vi "Initialize.vi"(8 "error in (no error)":errorcluster, 9 "Baud Rate":u32(ring)=9600 items=["9600"=9600, "38400"=38400, "57600"=57600, "19200"=19200], 11 "VISA resource name":refnum<visa-resource-name>) -> (0 "error out":errorcluster, 3 "VISA resource name out":refnum<visa-resource-name>)   [LabVIEW 2010, in "FEM-03.lvlib"]
doc: "Establishes communication with the instrument and optionally performs an instrument identification query and/or an instrument reset. It also places the instrument in a default state needed for other instrument driver operations. Therefore, call this VI before calling other instrument driver VIs for this instrument. Generally, you need to call the Initialize VI only once at the beginning of an application."
uses:
  FEM-03.lvlib
panel:
  # "(c) 2007 <Enter Company Name Here>.  ALL RIGHTS RESERVED."
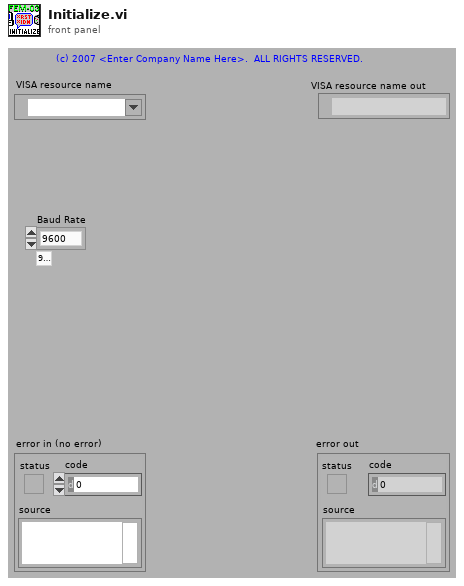
[diagram p1: front panel]
types:
  T1 = cluster{"Baud Rate":u32, "Parity":u16, "Data Bits":u16, "Stop Bits":u16, "Flow Control":u16}
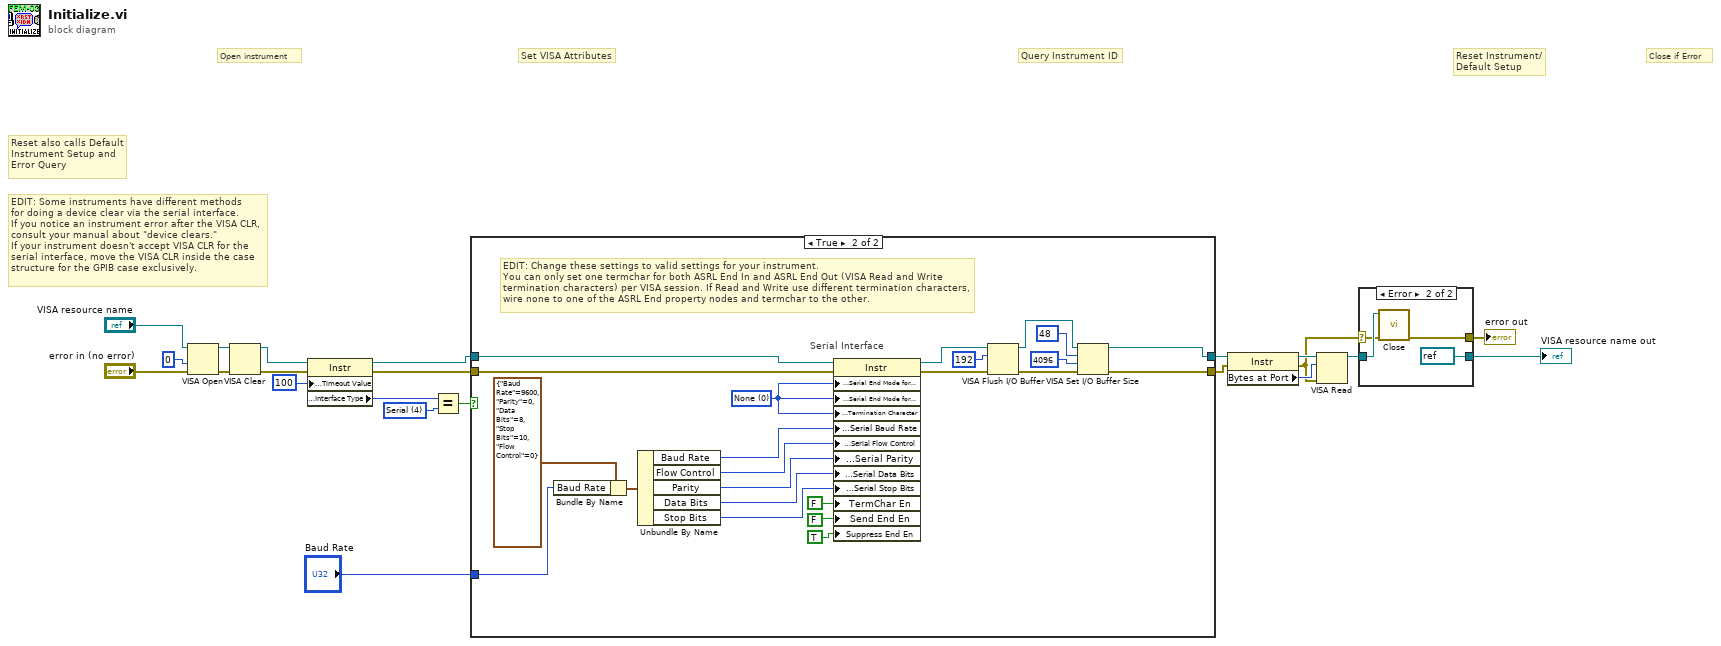
[diagram p0: block diagram]
diagram:
  w15 = u16 4 items=["GPIB"=1, "VXI"=2, "GPIB-VXI"=3, "Serial"=4, "PXI"=5, "TCPIP"=6, "USB"=7] ("Interface Information:Interface Type")
  # "Reset also calls Default Instrument Setup and Error Query"
  # "EDIT: Some instruments have different methods\nfor doing a device clear via the serial interface.  \nIf you notice an instrument error after the VISA CLR,\nconsult your manual about \"device clears.\"  \nIf your instrument doesn't accept VISA CLR for the\nserial interface, move the VISA CLR inside the case \nstructure for the GPIB case exclusively."
  # "Set VISA Attributes"
  # "Close if Error"
  # "Query Instrument ID"
  # "Reset Instrument/\nDefault Setup"
  # "Open instrument"
  n1 = VISA Open(access mode=u32 0, error in (no error)="error in (no error)", VISA resource name="VISA resource name") -> (VISA resource name=w13:refnum<visa-resource-name>, error out=w12:errorcluster)  [unwired: 2 in]
  n2 = VISA Clear(VISA resource name=w13, error in (no error)=w12) -> (VISA resource name out=w11:refnum<visa-resource-name>, error out=w10:errorcluster)
  n3 = property class="Instr"(reference=w11, error in=w10, "General Settings:Timeout Value"=u32 100) -> (reference out=w18:refnum<visa-resource-name>, error out=w17:errorcluster, "Interface Information:Interface Type"=w20:u16)
  n4 = Equal?(x=w20, y=w15) -> (x = y?=w16:bool)
  n5 = case shown="True" w16 {
    tunnel: [w23 w44] -> w6
    tunnel: [w24 w41] -> w3
    tunnel: w18 -> [w23 w46]
    tunnel: w17 -> [w24 w47]
    tunnel: "Baud Rate" -> [_ w25]
    frame False {
      # "EDIT: Remove interfaces not\nsupported by your instrument."
      # "GPIB, TCP/IP, and USB Interface"
    }
    frame True {
      w27 = u16 0 items=["None", "LastBit", "TermChar"] ("Serial Settings:Serial End Mode for Reads")
      # "EDIT: Change these settings to valid settings for your instrument.\nYou can only set one termchar for both ASRL End In and ASRL End Out (VISA Read and Write termination characters) per VISA session. If Read and Write use different termination characters, wire none to one of the ASRL End property nodes and termchar to the other."
      # "Serial Interface"
      n6 = Bundle By Name(cluster=T1 {"Baud Rate"=9600, "Parity"=0, "Data Bits"=8, "Stop Bits"=10, "Flow Control"=0} ("Serial Configuration"), "Baud Rate"=w25) -> (w26:T1)
      n7 = Unbundle By Name(w26) -> ("Baud Rate"=w36:u32, "Flow Control"=w32:u16, "Parity"=w34:u16, "Data Bits"=w35:u16, "Stop Bits"=w31:u16)
      n8 = property class="Instr"(reference=w46, error in=w47, "Serial Settings:Serial End Mode for Reads"=w27, "Serial Settings:Serial End Mode for Writes"=w27, "Message Based Settings:Termination Character"=w27, "Serial Settings:Serial Baud Rate"=w36, "Serial Settings:Serial Flow Control"=w32, "Serial Settings:Serial Parity"=w34, "Serial Settings:Serial Data Bits"=w35, "Serial Settings:Serial Stop Bits"=w31, "TermChar En"=FALSE ("Message Based Settings:Termination Character Enable"), "Send End En"=FALSE ("Message Based Settings:Send End Enable"), "Suppress End En"=TRUE ("Message Based Settings:Suppress End Enable")) -> (reference out=w40:refnum<visa-resource-name>, error out=w43:errorcluster)
      n9 = VISA Flush I/O Buffer(VISA resource name=w40, mask (16)=u16 192, error in (no error)=w43) -> (VISA resource name out=w45:refnum<visa-resource-name>, error out=w42:errorcluster)
      n10 = VISA Set I/O Buffer Size(VISA resource name=w45, mask (16)=u16 48, size (4096)=u32 4096 ("size (0)"), error in (no error)=w42) -> (VISA resource name out=w44:refnum<visa-resource-name>, error out=w41:errorcluster)
    }
  }
  n11 = property class="Instr"(reference=w6, error in=w3) -> (reference out=w5:refnum<visa-resource-name>, error out=w2:errorcluster, "Bytes at Port"=w4:u32)
  n12 = VISA Read(VISA resource name=w5, byte count=w4, error in (no error)=w2) -> (VISA resource name out=w7:refnum<visa-resource-name>)  [unwired: 3 out]
  n13 = case shown="Error" w2 {
    selector: w2 -> [w48 w51]
    tunnel: w7 -> [w49 w52]
    tunnel: [w49 refnum<visa-resource-name> refnum ("VISA resource name out")] -> w9
    tunnel: [w48 w53] -> w8
    frame No Error {
    }
    frame Error {
      n14 = call "Close.vi"("error in (no error)"=w51, "VISA resource name"=w52) -> ("error out"=w53:errorcluster)  [unwired: 9 in]
    }
  }
  "VISA resource name out" <- w9
  "error out" <- w8
